vi "TCP Loop.vi"(7 "TCP Exit":refnum<notifier>, 8 "error in":errorcluster, 10 "PLC Queue":refnum<queue>, 11 "TCP Queue":refnum<queue>) -> (0 "error out":errorcluster)   [LabVIEW 2015, in "TCP.lvlib"]
uses:
  TCP.lvlib
  support/Message Queue/Message Queue.lvlib
  <vilib>/ErrorRing/Error Ring.xnode
  TypeDefs/TCP Data.ctl
  PL Model/PL Model.lvlib
  <vilib>/Utility/error.llb/Error Cluster From Error Code.vi
  support/Message Queue/Message Cluster.ctl
panel:
  out "Message":string
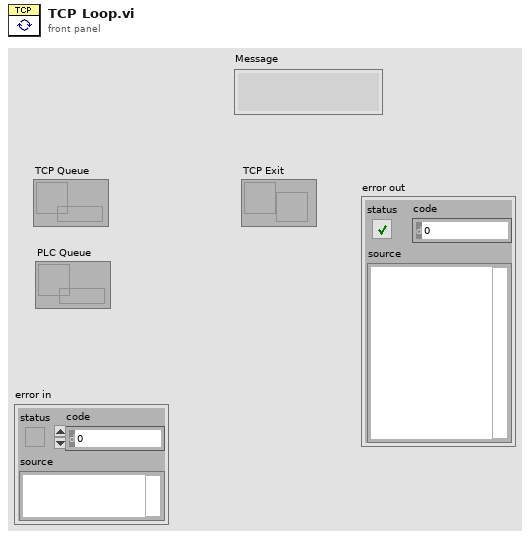
[diagram p1: front panel]
types:
  T1 = typedef "TCP.lvlib/TCP Data.ctl" = cluster{"Type":enum16{"Server", "Client"}, "IP":string, "Port":u16, "connection ID":refnum<k5>, "error":errorcluster, "Connected?":bool, "Data":string}
  T2 = enum16{"Standard", "Buffered", "CRLF", "Immediate"}
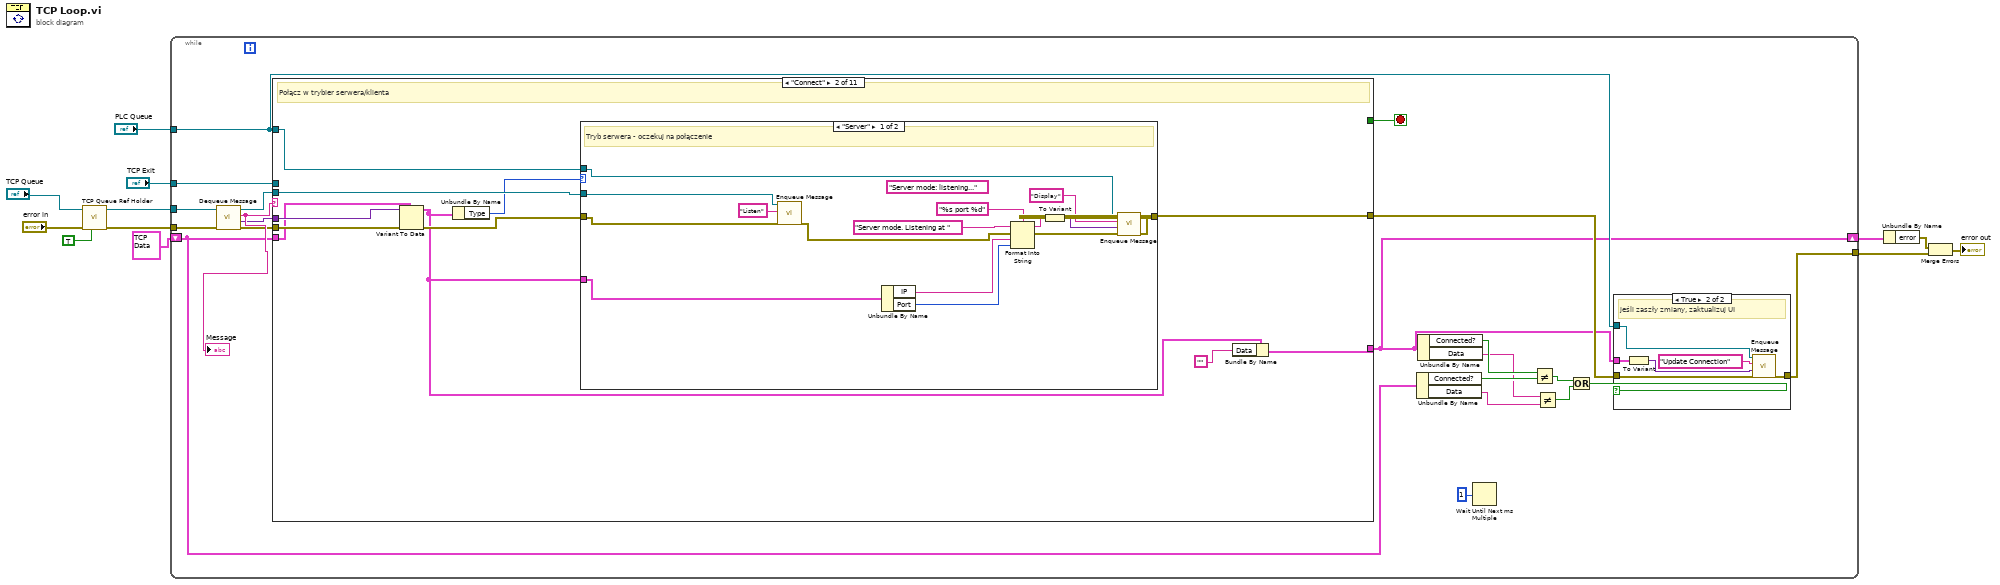
[diagram p0: block diagram]
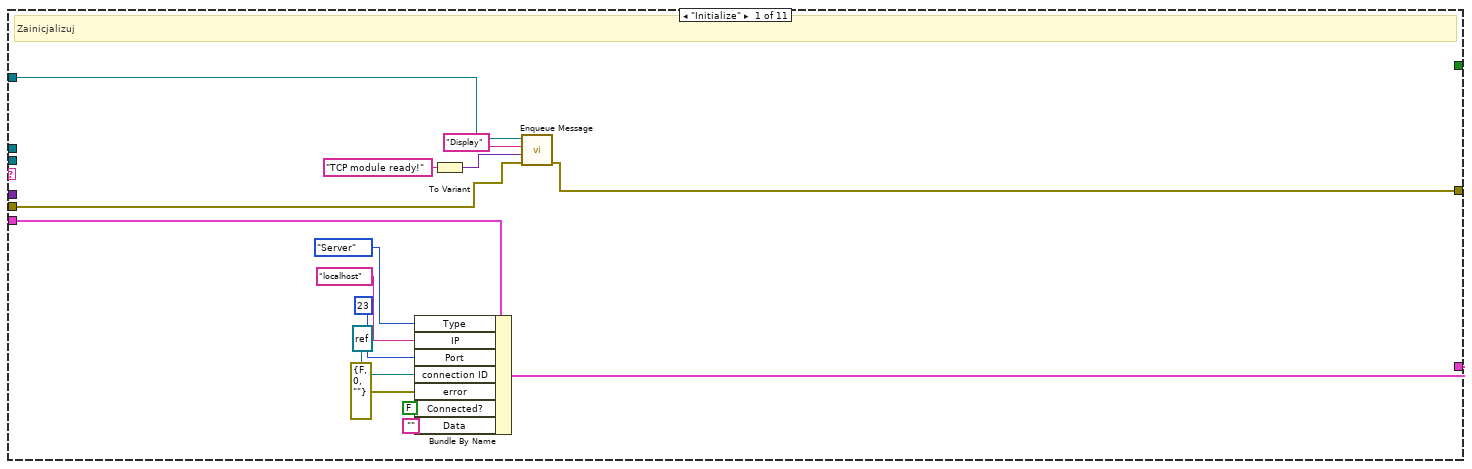
[diagram p3: hidden frame]
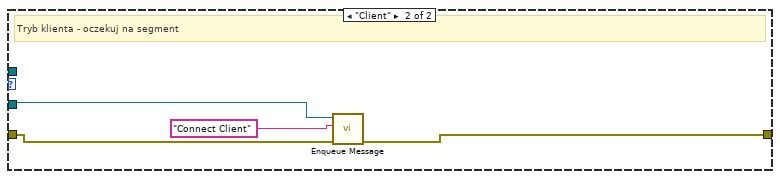
[diagram p4: hidden frame]
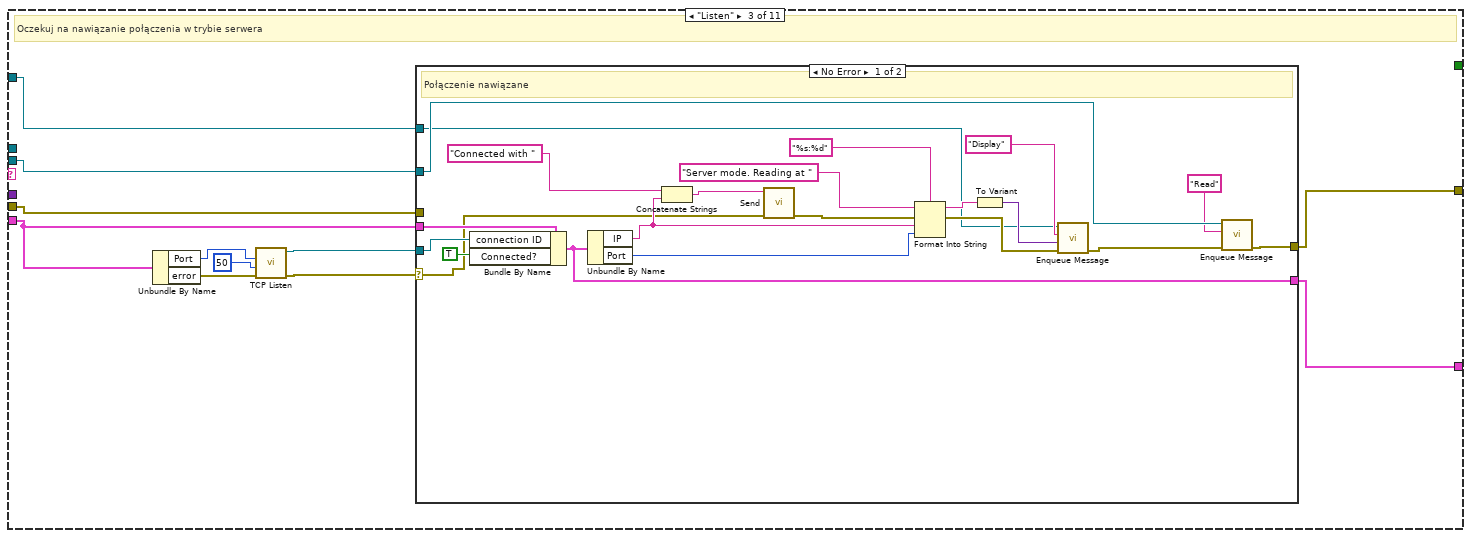
[diagram p5: hidden frame]
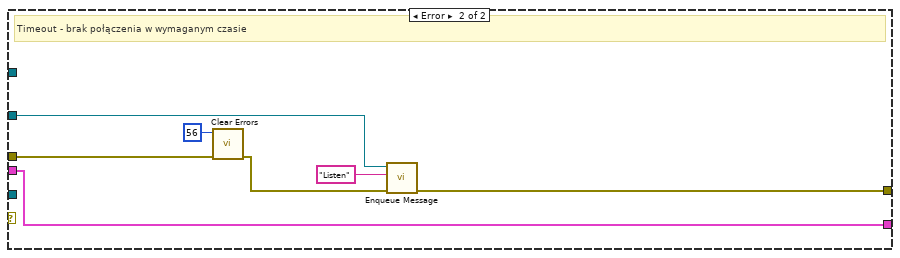
[diagram p6: hidden frame]
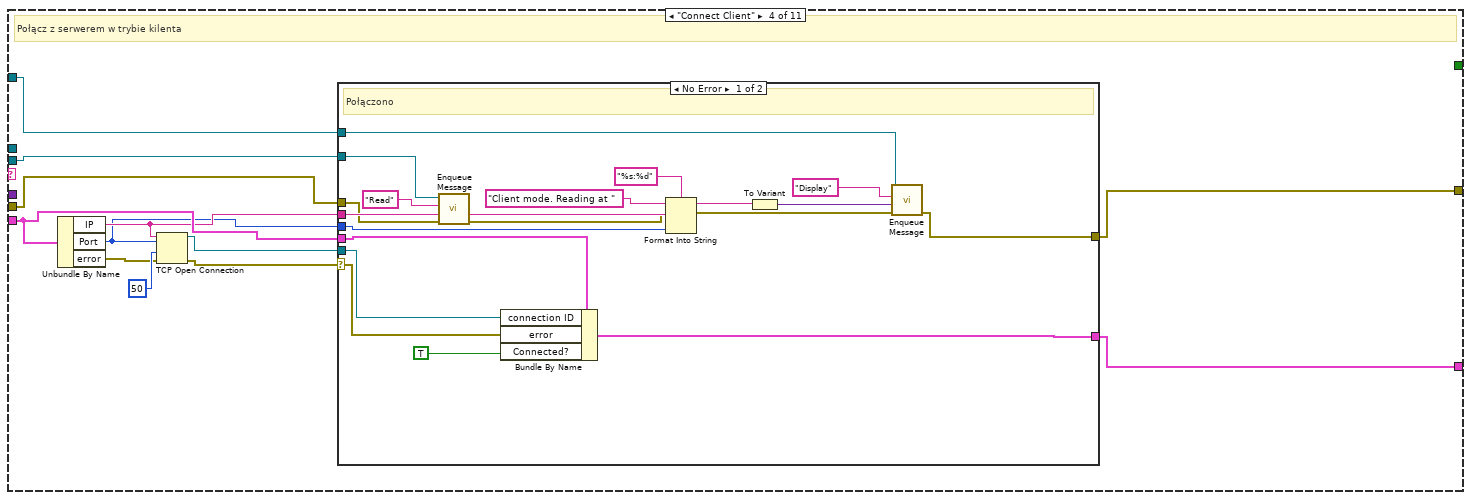
[diagram p7: hidden frame]
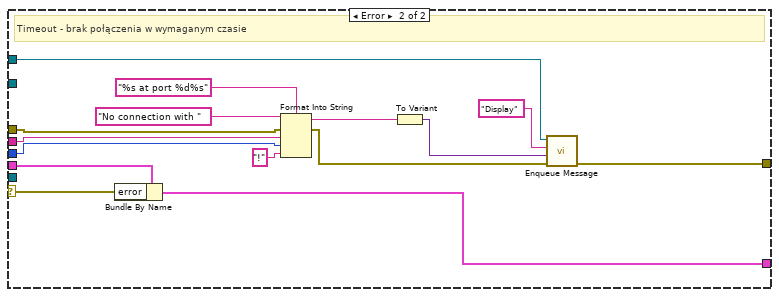
[diagram p8: hidden frame]
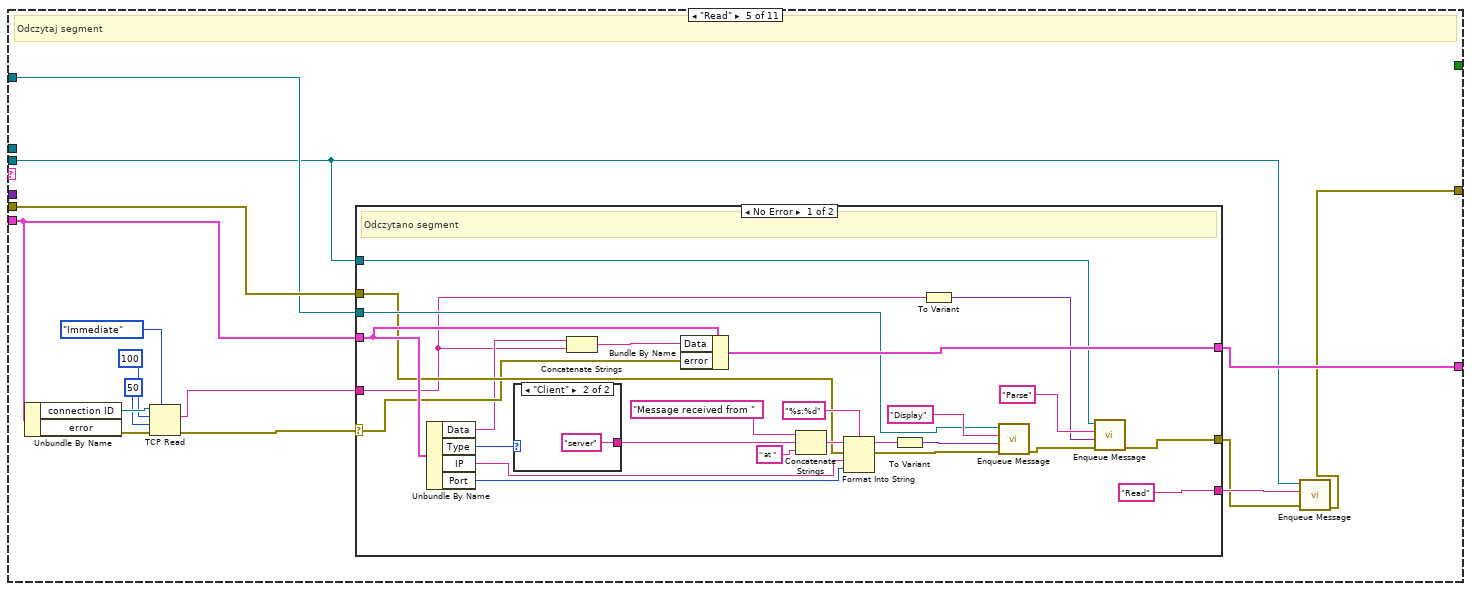
[diagram p9: hidden frame]
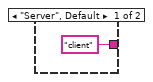
[diagram p10: hidden frame]
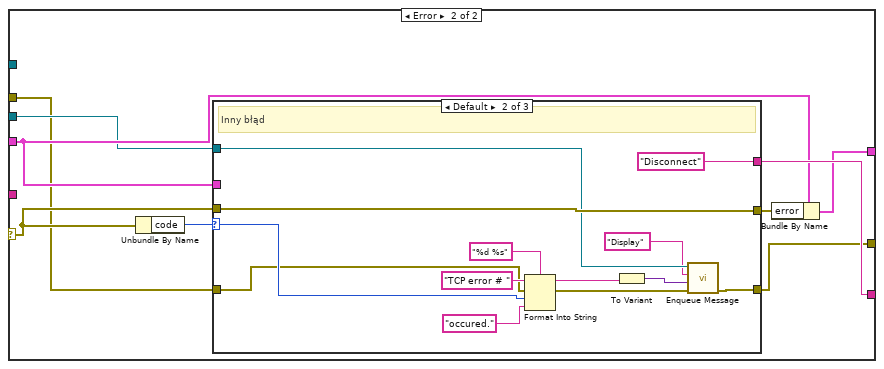
[diagram p11: hidden frame]
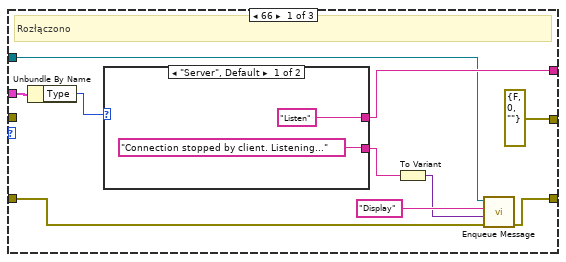
[diagram p12: hidden frame]
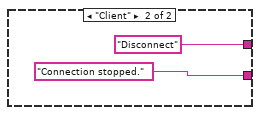
[diagram p13: hidden frame]
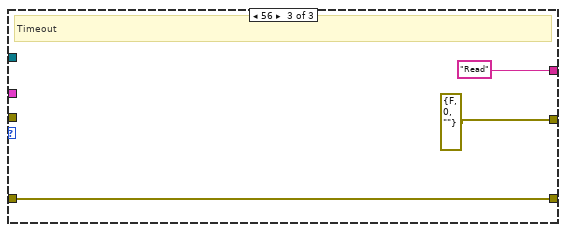
[diagram p14: hidden frame]
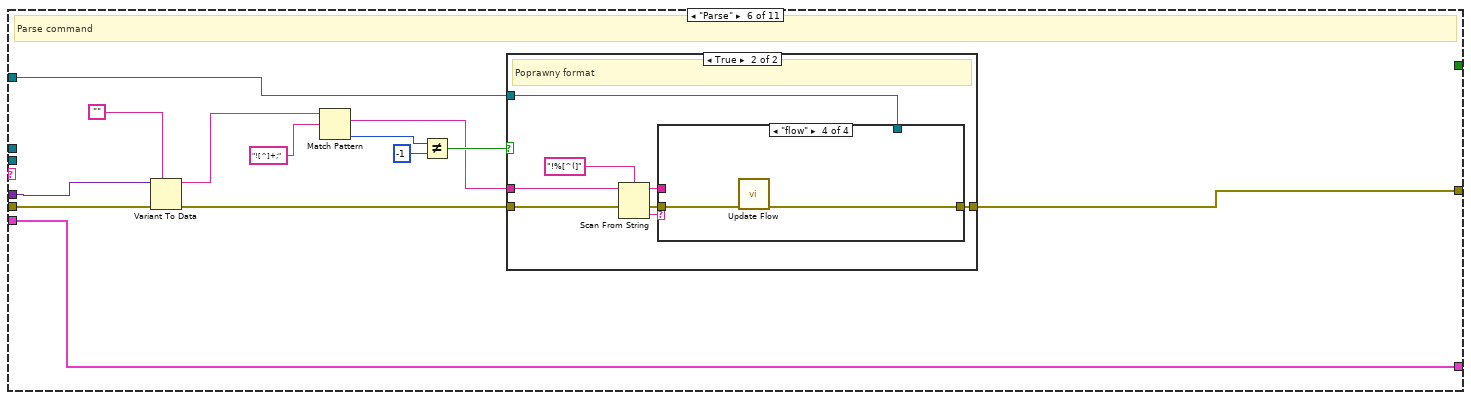
[diagram p15: hidden frame]
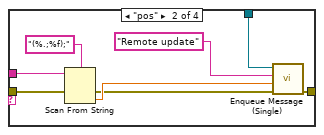
[diagram p18: hidden frame]
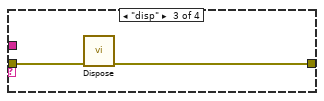
[diagram p19: hidden frame]
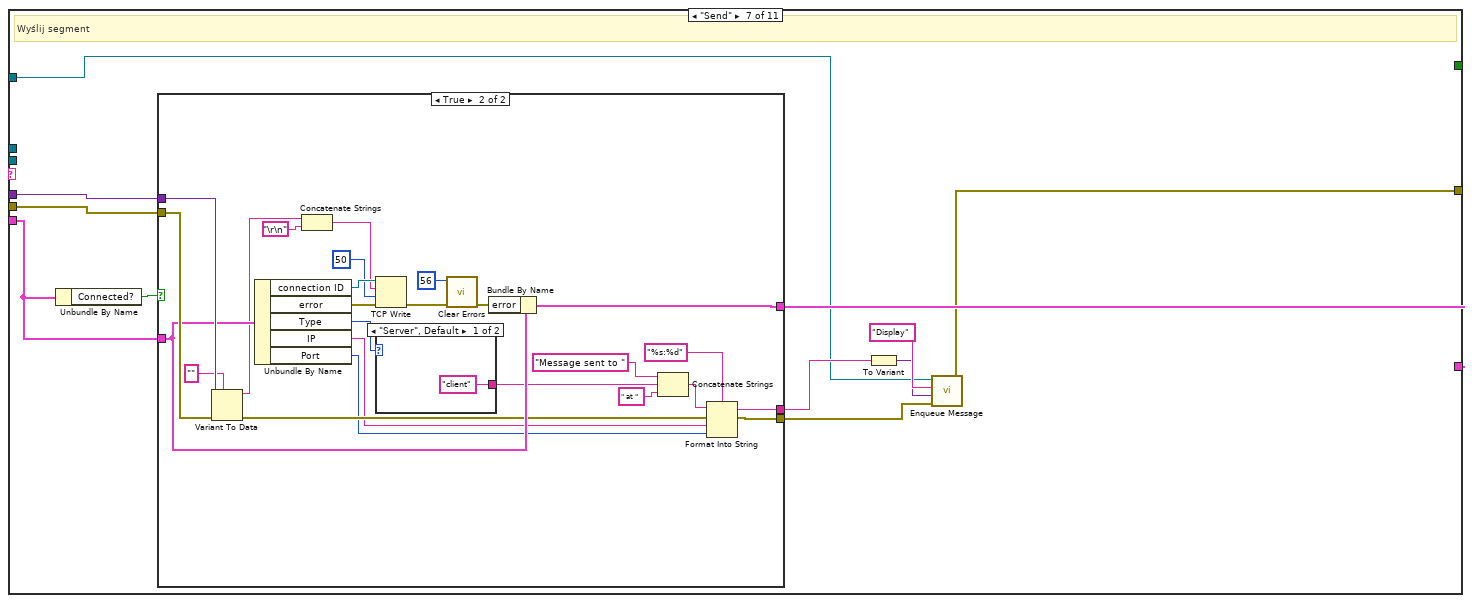
[diagram p20: hidden frame]
diagram:
  n1 = call "TCP Queue Ref Holder.vi"("Hold"=TRUE, "error in (no error)"="error in", "TCP Queue"="TCP Queue") -> ("error out"=w6:errorcluster, "Input Queue"=w8:refnum<queue>)  [unwired: 7 in]
  n2 = while {
    tunnel: w8 -> [w33]
    tunnel: w6 -> [w32]
    tunnel: [w24] -> w2
    tunnel: "TCP Exit" -> [w27]
    tunnel: "PLC Queue" -> [w15]
    shift-right: [w14] -> w4
    shift-left: T1 {"Type"=enum."Server", "IP"="", "Port"=0, "connection ID"=refnum, "error"={"status"=FALSE, "code"=0, "source"=""}, "Connected?"=FALSE, "Data"=""} ("TCP Data") -> [w23]
    stop <- w28 stop-if-true
    n3 = call "Dequeue Message.vi"("error in (no error)"=w32, "Message Queue"=w33) -> ("error out"=w30:errorcluster, "Message Data"=w26:variant, "Message"=w31:string, "dup Message Queue"=w29:refnum<queue>)  [unwired: 6 in]
    "Message" <- w31
    n4 = case shown="\"Connect\"" w31 {
      selector: w31 -> [_ _ _ _ _ _ _ _ _ w359 _]
      tunnel: w30 -> [w51 w65 w87 w129 w176 w263 w298 w341 w355 _ w370]
      tunnel: [w50 w64 w91 w128 w173 w254 w291 w343 w351 w358 w371] -> w25
      tunnel: w29 -> [_ w66 w92 w130 w171 _ _ w340 w354 _ _]
      tunnel: [_ _ _ _ _ _ _ _ TRUE TRUE _] -> w28
      tunnel: w27 -> [_ _ _ _ _ _ _ _ w349 _ _]
      tunnel: w15 -> [w52 w60 w86 w127 w172 w253 w290 w342 _ _ _]
      tunnel: w23 -> [w49 w62 w89 w132 w177 w260 w289 w339 w346 w357 w369]
      tunnel: [w48 w61 w88 w131 w175 w260 w296 w344 w345 w357 w369] -> w14
      tunnel: w26 -> [_ w63 _ _ _ w265 w297 _ _ _ _]
      frame "Initialize" {
        # "Zainicjalizuj"
        n5 = Bundle By Name(cluster=w49, "Type"=enum16{"Server", "Client"}."Server", "IP"="localhost", "Port"=u16 23, "connection ID"=refnum<k5> refnum, "error"=errorcluster {"status"=FALSE, "code"=0, "source"=""}, "Connected?"=FALSE, "Data"="") -> (w48:T1)
        n6 = To Variant(anything="TCP module ready!" ("Message")) -> (Variant=w53:variant)
        n7 = call-poly "Enqueue Message.vi"("error in (no error)"=w51, "Message Data"=w53, "Message"="Display", "Message Queue"=w52) -> ("error out"=w50:errorcluster)  [unwired: 6 in, 1 out]
      }
      frame "Connect" {
        # "Połącz w trybier serwera/klienta"
        n8 = Variant To Data(error in=w65, type=w62, Variant=w63) -> (data=w56:T1, error out=w59:errorcluster)
        n9 = Unbundle By Name(w56) -> ("Type"=w58:enum16{"Server", "Client"})
        n10 = case shown="\"Server\"" w58 {
          tunnel: w66 -> [w80 w85]
          tunnel: w59 -> [w69 w83]
          tunnel: [w78 w82] -> w64
          tunnel: w60 -> [w72 _]
          tunnel: w56 -> [w70 _]
          frame "Server" {
            (unwired) "Server mode: listening..." ("Message")
            # "Tryb serwera - oczekuj na połączenie"
            n11 = call-poly "Enqueue Message.vi"("error in (no error)"=w69, "Message"="Listen", "Message Queue"=w80) -> ("error out"=w68:errorcluster)  [unwired: 7 in, 1 out]
            n12 = Unbundle By Name(w70) -> ("IP"=w71:string, "Port"=w73:u16)
            n13 = Format Into String(format string="%s port %d", initial string="Server mode. Listening at " ("Message"), error in=w68, w71, w73) -> (resulting string=w67:string, error out=w74:errorcluster)
            n14 = To Variant(anything=w67) -> (Variant=w77:variant)
            n15 = call-poly "Enqueue Message.vi"("error in (no error)"=w74, "Message Data"=w77, "Message"="Display", "Message Queue"=w72) -> ("error out"=w78:errorcluster)  [unwired: 6 in, 1 out]
          }
          frame "Client" {
            # "Tryb klienta - oczekuj na segment"
            n16 = call-poly "Enqueue Message.vi"("error in (no error)"=w83, "Message"="Connect Client", "Message Queue"=w85) -> ("error out"=w82:errorcluster)  [unwired: 7 in, 1 out]
          }
        }
        n17 = Bundle By Name(cluster=w56, "Data"="") -> (w61:T1)
      }
      frame "Listen" {
        # "Oczekuj na nawiązanie połączenia w trybie serwera"
        n18 = Unbundle By Name(w89) -> ("Port"=w96:u16, "error"=w94:errorcluster)
        n19 = call <vilib>:"TCP Listen.vi"("error in (no error)"=w94, "timeout ms (wait forever: -1)"=50, "port"=w96) -> ("error out"=w93:errorcluster, "connection ID"=w90:refnum<k5>)  [unwired: 4 in, 3 out]
        n20 = case shown="No Error" w93 {
          selector: w93 -> [w100 _]
          tunnel: w92 -> [w117 w124]
          tunnel: [w97 w119] -> w91
          tunnel: w90 -> [w114 _]
          tunnel: w89 -> [w115 w118]
          tunnel: [w101 w118] -> w88
          tunnel: w87 -> [_ w121]
          tunnel: w86 -> [w106 _]
          frame No Error {
            # "Połączenie nawiązane"
            n21 = Bundle By Name(cluster=w115, "connection ID"=w114, "Connected?"=TRUE) -> (w101:T1)
            n22 = Unbundle By Name(w101) -> ("IP"=w102:string, "Port"=w105:u16)
            n23 = Concatenate Strings("Connected with " ("string"), w102) -> (w104:string)
            n24 = call "Send.vi"("error in"=w100, "Data"=w104) -> ("error out"=w99:errorcluster)  [unwired: 9 in]
            n25 = Format Into String(format string="%s:%d", initial string="Server mode. Reading at " ("Message"), error in=w99, w102, w105) -> (resulting string=w109:string, error out=w110:errorcluster)
            n26 = To Variant(anything=w109) -> (Variant=w108:variant)
            n27 = call-poly "Enqueue Message.vi"("error in (no error)"=w110, "Message Data"=w108, "Message"="Display", "Message Queue"=w106) -> ("error out"=w98:errorcluster)  [unwired: 6 in, 1 out]
            n28 = call-poly "Enqueue Message.vi"("error in (no error)"=w98, "Message"="Read", "Message Queue"=w117) -> ("error out"=w97:errorcluster)  [unwired: 7 in, 1 out]
          }
          frame Error {
            # "Timeout - brak połączenia w wymaganym czasie"
            n29 = call <vilib>:"Clear Errors.vi"("error in (no error)"=w121, "specific error code to clear (0: all)"=56) -> ("error out"=w122:errorcluster)  [unwired: 4 in, 1 out]
            n30 = call-poly "Enqueue Message.vi"("error in (no error)"=w122, "Message"="Listen", "Message Queue"=w124) -> ("error out"=w119:errorcluster)  [unwired: 7 in, 1 out]
          }
        }
      }
      frame "Connect Client" {
        # "Połącz z serwerem w trybie kilenta"
        n31 = Unbundle By Name(w132) -> ("IP"=w126:string, "Port"=w125:u16, "error"=w135:errorcluster)
        n32 = TCP Open Connection(address=w126, remote port or service name=w125, timeout ms (60000)=50, error in (no error)=w135) -> (connection ID=w133:refnum<k5>, error out=w134:errorcluster)  [unwired: 1 in]
        n33 = case shown="No Error" w134 {
          selector: w134 -> [w137 w159]
          tunnel: [w152 w169] -> w131
          tunnel: w133 -> [w154 _]
          tunnel: w132 -> [w155 w170]
          tunnel: w129 -> [w138 w158]
          tunnel: w130 -> [w151 _]
          tunnel: [w147 w165] -> w128
          tunnel: w127 -> [w140 w166]
          tunnel: w126 -> [w142 w162]
          tunnel: w125 -> [w141 w161]
          frame No Error {
            # "Połączono"
            n34 = call-poly "Enqueue Message.vi"("error in (no error)"=w138, "Message"="Read", "Message Queue"=w151) -> ("error out"=w139:errorcluster)  [unwired: 7 in, 1 out]
            n35 = Bundle By Name(cluster=w155, "connection ID"=w154, "error"=w137, "Connected?"=TRUE) -> (w152:T1)
            n36 = Format Into String(format string="%s:%d", initial string="Client mode. Reading at " ("Message"), error in=w139, w142, w141) -> (resulting string=w144:string, error out=w143:errorcluster)
            n37 = To Variant(anything=w144) -> (Variant=w148:variant)
            n38 = call-poly "Enqueue Message.vi"("error in (no error)"=w143, "Message Data"=w148, "Message"="Display", "Message Queue"=w140) -> ("error out"=w147:errorcluster)  [unwired: 6 in, 1 out]
          }
          frame Error {
            # "Timeout - brak połączenia w wymaganym czasie"
            n39 = Bundle By Name(cluster=w170, "error"=w159) -> (w169:T1)
            n40 = Format Into String(format string="%s at port %d%s", initial string="No connection with " ("Message"), error in=w158, w162, w161, "!" ("input 3")) -> (resulting string=w160:string, error out=w157:errorcluster)
            n41 = To Variant(anything=w160) -> (Variant=w167:variant)
            n42 = call-poly "Enqueue Message.vi"("error in (no error)"=w157, "Message Data"=w167, "Message"="Display", "Message Queue"=w166) -> ("error out"=w165:errorcluster)  [unwired: 6 in, 1 out]
          }
        }
      }
      frame "Read" {
        # "Odczytaj segment"
        n43 = Unbundle By Name(w177) -> ("connection ID"=w185:refnum<k5>, "error"=w182:errorcluster)
        n44 = TCP Read(connection ID=w185, bytes to read=100, error in (no error)=w182, 7:T2."Immediate" ("mode (standard)"), 9:50 ("timeout ms (25000)")) -> (data out=w178:string, error out=w180:errorcluster)  [unwired: 1 out]
        n45 = case shown="No Error" w180 {
          selector: w180 -> [w193 w220]
          tunnel: [w210 w219] -> w175
          tunnel: ["Read" ("Message") w221] -> w179
          tunnel: w178 -> [w186 _]
          tunnel: w177 -> [w209 w217]
          tunnel: w172 -> [w199 w216]
          tunnel: w176 -> [w196 w215]
          tunnel: [w191 w214] -> w174
          tunnel: w171 -> [w187 _]
          frame No Error {
            # "Odczytano segment"
            n46 = Unbundle By Name(w209) -> ("Data"=w189:string, "Type"=w198:enum16{"Server", "Client"}, "IP"=w194:string, "Port"=w197:u16)
            n47 = case shown="\"Client\"" w198 {
              tunnel: ["client" ("Message") "server" ("f")] -> w195
              frame "Server", Default {
              }
              frame "Client" {
              }
            }
            n48 = Concatenate Strings(w189, w186) -> (w208:string)
            n49 = Bundle By Name(cluster=w209, "Data"=w208, "error"=w193) -> (w210:T1)
            n50 = Concatenate Strings("Message received from " ("Message"), w195, " at " ("string")) -> (w202:string)
            n51 = Format Into String(format string="%s:%d", initial string=w202, error in=w196, w194, w197) -> (resulting string=w205:string, error out=w204:errorcluster)
            n52 = To Variant(anything=w205) -> (Variant=w206:variant)
            n53 = To Variant(anything=w186) -> (Variant=w188:variant)
            n54 = call-poly "Enqueue Message.vi"("error in (no error)"=w204, "Message Data"=w206, "Message"="Display", "Message Queue"=w199) -> ("error out"=w192:errorcluster)  [unwired: 6 in, 1 out]
            n55 = call-poly "Enqueue Message.vi"("error in (no error)"=w192, "Message Data"=w188, "Message"="Parse", "Message Queue"=w187) -> ("error out"=w191:errorcluster)  [unwired: 6 in, 1 out]
          }
          frame Error {
            n56 = Unbundle By Name(w220) -> ("code"=w222:i32)
            n57 = case shown="Default" w222 {
              selector: w222 -> [_ w242 _]
              tunnel: [w229 "Disconnect" ("Message") "Read" ("Message")] -> w221
              tunnel: w220 -> [_ w249 _]
              tunnel: [errorcluster {"status"=FALSE, "code"=0, "source"=""} ("error") w249 errorcluster {"status"=FALSE, "code"=0, "source"=""} ("error")] -> w218
              tunnel: w217 -> [w231 _ _]
              tunnel: w216 -> [w228 w247 _]
              tunnel: w215 -> [w226 w238 w250]
              tunnel: [w227 w246 w250] -> w214
              frame 66 {
                # "Rozłączono"
                n58 = Unbundle By Name(w231) -> ("Type"=w230:enum16{"Server", "Client"})
                n59 = case shown="\"Server\", Default" w230 {
                  tunnel: ["Listen" ("Message") "Disconnect" ("Message")] -> w229
                  tunnel: ["Connection stopped by client. Listening..." ("Message") "Connection stopped." ("Message")] -> w224
                  frame "Server", Default {
                  }
                  frame "Client" {
                  }
                }
                n60 = To Variant(anything=w224) -> (Variant=w223:variant)
                n61 = call-poly "Enqueue Message.vi"("error in (no error)"=w226, "Message Data"=w223, "Message"="Display", "Message Queue"=w228) -> ("error out"=w227:errorcluster)  [unwired: 6 in, 1 out]
              }
              frame Default {
                # "Inny błąd"
                n62 = Format Into String(format string="%d %s", initial string="TCP error # " ("Message"), error in=w238, w242, "occured." ("input 2")) -> (resulting string=w240:string, error out=w237:errorcluster)
                n63 = To Variant(anything=w240) -> (Variant=w239:variant)
                n64 = call-poly "Enqueue Message.vi"("error in (no error)"=w237, "Message Data"=w239, "Message"="Display", "Message Queue"=w247) -> ("error out"=w246:errorcluster)  [unwired: 6 in, 1 out]
              }
              frame 56 {
                # "Timeout"
              }
            }
            n65 = Bundle By Name(cluster=w217, "error"=w218) -> (w219:T1)
          }
        }
        n66 = call-poly "Enqueue Message.vi"("error in (no error)"=w174, "Message"=w179, "Message Queue"=w171) -> ("error out"=w173:errorcluster)  [unwired: 7 in, 1 out]
      }
      frame "Parse" {
        # "Parse command"
        n67 = Variant To Data(error in=w263, type="", Variant=w265) -> (data=w262:string, error out=w255:errorcluster)
        n68 = Match Pattern(string=w262, regular expression="![^]+;") -> (match substring=w256:string, offset past match=w259:i32)  [unwired: 1 in, 2 out]
        n69 = Not Equal?(x=w259, y=-1) -> (x != y?=w257:bool)
        n70 = case shown="True" w257 {
          tunnel: w256 -> [_ w274]
          tunnel: w255 -> [w266 w273]
          tunnel: [w266 w269] -> w254
          tunnel: w253 -> [_ w268]
          frame False {
            # "Zła postać"
          }
          frame True {
            # "Poprawny format"
            n71 = Scan From String(format string="!%[^(]", input string=w274, error in=w273) -> (remaining string=w267:string, error out=w270:errorcluster, output 1=w271:string)  [unwired: 2 in, 1 out]
            n72 = case shown="\"flow\"" w271 {
              tunnel: w270 -> [w275 w278 w285 w287]
              tunnel: [w275 w282 w284 w286] -> w269
              tunnel: w268 -> [_ w283 _ _]
              tunnel: w267 -> [_ w279 _ _]
              frame Default {
              }
              frame "pos" {
                n73 = Scan From String(format string="(%.;%f);", input string=w279, error in=w278) -> (error out=w276:errorcluster, output 1=w277:dbl)  [unwired: 2 in, 2 out]
                n74 = call "Enqueue Message (Single).vi"("error in (no error)"=w276, "Message Data"=w277, "Message"="Remote update", "Message Queue"=w283) -> ("error out"=w282:errorcluster)  [unwired: 6 in, 1 out]
              }
              frame "disp" {
                n75 = call "Dispose.vi"("error in (no error)"=w285) -> ("error out"=w284:errorcluster)  [unwired: 10 in]
              }
              frame "flow" {
                n76 = call "Update Flow.vi"("error in (no error)"=w287) -> ("error out"=w286:errorcluster)  [unwired: 10 in]
              }
            }
          }
        }
      }
      frame "Send" {
        # "Wyślij segment"
        n77 = Unbundle By Name(w289) -> ("Connected?"=w288:bool)
        n78 = case shown="True" w288 {
          tunnel: w298 -> [w300 w324]
          tunnel: w297 -> [_ w323]
          tunnel: w289 -> [w299 w321]
          tunnel: [w299 w302] -> w296
          tunnel: ["No connection - data not sent!" w316] -> w293
          tunnel: [w300 w315] -> w292
          frame False {
          }
          frame True {
            n79 = Variant To Data(error in=w324, type="", Variant=w323) -> (data=w304:string, error out=w314:errorcluster)
            n80 = Unbundle By Name(w321) -> ("connection ID"=w326:refnum<k5>, "error"=w325:errorcluster, "Type"=w311:enum16{"Server", "Client"}, "IP"=w305:string, "Port"=w308:u16)
            n81 = Concatenate Strings(w304, "\r\n") -> (w306:string)
            n82 = TCP Write(connection ID=w326, data in=w306, error in (no error)=w325, 9:50 ("timeout ms (25000)")) -> (error out=w320:errorcluster)  [unwired: 2 out]
            n83 = case shown="\"Server\", Default" w311 {
              tunnel: ["client" ("Message") "server" ("f")] -> w310
              frame "Server", Default {
              }
              frame "Client" {
              }
            }
            n84 = call <vilib>:"Clear Errors.vi"("error in (no error)"=w320, "specific error code to clear (0: all)"=56) -> ("error out"=w319:errorcluster)  [unwired: 4 in, 1 out]
            n85 = Bundle By Name(cluster=w321, "error"=w319) -> (w302:T1)
            n86 = Concatenate Strings("Message sent to " ("Message"), w310, " at " ("string")) -> (w312:string)
            n87 = Format Into String(format string="%s:%d", initial string=w312, error in=w314, w305, w308) -> (resulting string=w316:string, error out=w315:errorcluster)
          }
        }
        n88 = To Variant(anything=w293) -> (Variant=w294:variant)
        n89 = call-poly "Enqueue Message.vi"("error in (no error)"=w292, "Message Data"=w294, "Message"="Display", "Message Queue"=w290) -> ("error out"=w291:errorcluster)  [unwired: 6 in, 1 out]
      }
      frame "Disconnect" {
        # "Rozłącz"
        n90 = Unbundle By Name(w339) -> ("connection ID"=w338:refnum<k5>, "error"=w332:errorcluster)
        n91 = TCP Close Connection(connection ID=w338, error in (no error)=w332) -> (error out=w331:errorcluster)  [unwired: 1 in, 1 out]
        n92 = Flush Queue(queue=w340, error in (no error)=w341) -> (error out=w329:errorcluster)  [unwired: 2 out]
        n93 = call <vilib>:"Clear Errors.vi"("error in (no error)"=w331) -> ("error out"=w330:errorcluster)  [unwired: 5 in, 1 out]
        n94 = Bundle By Name(cluster=w339, "connection ID"=refnum<k5> refnum, "error"=w330, "Connected?"=FALSE) -> (w344:T1)
        n95 = To Variant(anything="Connection closed." ("Message")) -> (Variant=w334:variant)
        n96 = call-poly "Enqueue Message.vi"("error in (no error)"=w329, "Message Data"=w334, "Message"="Display", "Message Queue"=w342) -> ("error out"=w343:errorcluster)  [unwired: 6 in, 1 out]
      }
      frame "Exit" {
        # "Zamknij moduł TCP"
        n97 = Release Queue(queue=w354, force destroy? (F)=TRUE, error in (no error)=w355) -> (error out=w352:errorcluster)  [unwired: 2 out]
        n98 = Send Notification(notification=TRUE ("force destroy? (F)"), notifier=w349, error in (no error)=w352) -> (error out=w351:errorcluster)  [unwired: 1 out]
        n99 = Bundle By Name(cluster=w346, "Connected?"=FALSE) -> (w345:T1)
      }
      frame Default {
        # "Błędna instrukcja"
        n100 = xnode "Error Ring"("parameter 0"=w359) -> ("error out"=w358:errorcluster)
      }
      frame "Say goodbye" {
        # "Wyślij informację o zakończeniu"
        n101 = Unbundle By Name(w369) -> ("Connected?"=w367:bool, "IP"=w368:string)
        n102 = case shown="True" w367 {
          tunnel: [w372 w377] -> w371
          tunnel: w370 -> [w372 w376]
          tunnel: w368 -> [_ w374]
          frame False {
          }
          frame True {
            n103 = Concatenate Strings("Disconnected with " ("string"), w374) -> (w373:string)
            n104 = call "Send.vi"("error in"=w376, "Data"=w373) -> ("error out"=w377:errorcluster)  [unwired: 9 in]
          }
        }
      }
    }
    n105 = Unbundle By Name(w23) -> ("Connected?"=w21:bool, "Data"=w19:string)
    n106 = Unbundle By Name(w14) -> ("Connected?"=w22:bool, "Data"=w20:string)
    n107 = Wait Until Next ms Multiple(millisecond multiple=u32 1) -> ()  [unwired: 1 out]
    n108 = Not Equal?(x=w22, y=w21) -> (x != y?=w18:bool)
    n109 = Not Equal?(x=w20, y=w19) -> (x != y?=w17:bool)
    n110 = Or(x=w18, y=w17) -> (x .or. y?=w16:bool)
    n111 = case shown="True" w16 {
      tunnel: w25 -> [w34 w40]
      tunnel: [w34 w39] -> w24
      tunnel: w15 -> [_ w38]
      tunnel: w14 -> [_ w36]
      frame False {
      }
      frame True {
        # "jeśli zaszły zmiany, zaktualizuj UI"
        n112 = To Variant(anything=w36) -> (Variant=w35:variant)
        n113 = call-poly "Enqueue Message.vi"("error in (no error)"=w40, "Message Data"=w35, "Message"="Update Connection", "Message Queue"=w38) -> ("error out"=w39:errorcluster)  [unwired: 6 in, 1 out]
      }
    }
  }
  n114 = Unbundle By Name(w4) -> ("error"=w3:errorcluster)
  n115 = Merge Errors(w3, w2) -> (→"error out":errorcluster)
